vi "新旧坐标系四点计算旋转角度.vi"(1 "新Point2":T2={"X"=100.0, "Y"=0.0, "Z"=99.0}, 2 "新Point1":T2, 3 "旧Point2":T2={"X"=0.0, "Y"=100.0, "Z"=0.0}, 4 "旧Point1":T2) -> (0 "新旧原点和旋转角度":T1 {"Rotation" format="%.2f"})   [LabVIEW 2014]
uses:
  Controls/XYZPos.ctl
panel:
  out "deg2":dbl
  out "deg1":dbl
  out "deg":dbl
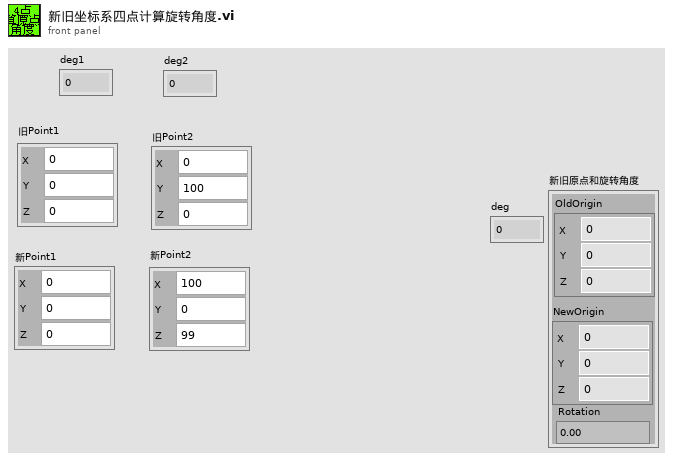
[diagram p1: front panel]
types:
  T1 = typedef "新旧原点和旋转角度.ctl" = cluster{"OldOrigin":T2, "NewOrigin":T2, "Rotation":dbl}
  T2 = typedef "XYZPos.ctl" = cluster{"X":dbl, "Y":dbl, "Z":dbl}
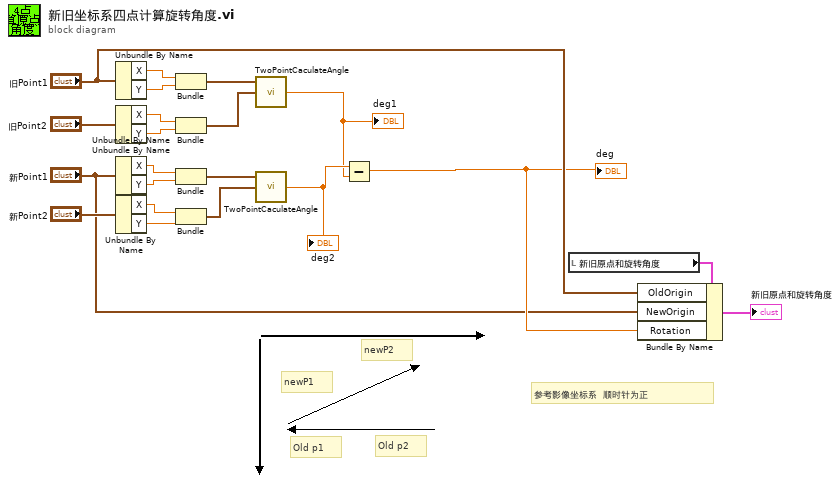
[diagram p0: block diagram]
diagram:
  # "参考影像坐标系  顺时针为正"
  # "newP2"
  # "newP1"
  # "Old p2"
  # "Old p1"
  n1 = Unbundle By Name("旧Point1") -> ("X"=w17:dbl, "Y"=w16:dbl)
  n2 = Unbundle By Name("旧Point2") -> ("X"=w14:dbl, "Y"=w15:dbl)
  n3 = Unbundle By Name("新Point1") -> ("X"=w20:dbl, "Y"=w21:dbl)
  n4 = Unbundle By Name("新Point2") -> ("X"=w19:dbl, "Y"=w18:dbl)
  n5 = Bundle("X"=w17, "Y"=w16) -> (w9:cluster{"X":dbl, "Y":dbl})  [unwired: 1 in]
  n6 = Bundle("X"=w14, "Y"=w15) -> (w8:cluster{"X":dbl, "Y":dbl})  [unwired: 1 in]
  n7 = Bundle("X"=w20, "Y"=w21) -> (w7:cluster{"X":dbl, "Y":dbl})  [unwired: 1 in]
  n8 = Bundle("X"=w19, "Y"=w18) -> (w6:cluster{"X":dbl, "Y":dbl})  [unwired: 1 in]
  n9 = call "TwoPointCaculateAngle.vi"("Point2"=w8, "Point1"=w9) -> ("角度"=w3:dbl)  [unwired: 1 in]
  "deg1" <- w3
  n10 = call "TwoPointCaculateAngle.vi"("Point2"=w6, "Point1"=w7) -> ("角度"=w4:dbl)  [unwired: 1 in]
  "deg2" <- w4
  n11 = Subtract(x=w4, y=w3) -> (x-y=w2:dbl)
  "deg" <- w2
  n12 = local read "新旧原点和旋转角度"() -> (w12:T1)
  n13 = Bundle By Name(cluster=w12, "OldOrigin"="旧Point1", "NewOrigin"="新Point1", "Rotation"=w2) -> (→"新旧原点和旋转角度":T1)
